vi "HP4284A_CommandsGlobal.vi"() -> ()   [LabVIEW 2018, in "HP4284A.lvclass"]
uses:
  HP4284A.lvclass
panel:
  in  "HP 4284A GPIB Setup":T1={"Instrument name"="HP 4284A", "Instrument type"=1, "Command \"Initialise LCR\""="CORR:LENG 2M;:CORR:METH SING;:CORR:OPEN:STAT %s;:CORR:SHORT:STAT %s;:CORR:LOAD:STAT OFF;:CORR:LOAD:TYPE CPD;:CORR:USE 0%.;;:FREQ %fHZ;:VOLT %fV;:AMPL:ALC OFF%.;;:FUNC:IMP:RANG 100000OHM;:FUNC:IMP:RANG:AUTO ON;:FUNC:IMP %s;:DISP:PAGE MEAS;:INIT:CONT OFF;:TRIG:SOUR INT;:TRIG:DEL 2.0;:APER MEDIUM,4", "Command \"OC Trim\""="CORR:OPEN;", "Command \"LCR Readout\""="TRIG:IMM;:FETC?"} {"Instrument type" items=["Supply", "LCR"]}
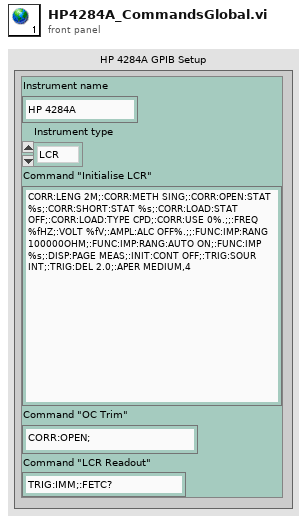
[diagram p1: front panel]
types:
  T1 = cluster{"Instrument name":string, "Instrument type":u16, "Command \"Initialise LCR\"":string, "Command \"OC Trim\"":string, "Command \"LCR Readout\"":string}
diagram:
